vi "generate_zernike_tilt_vectors.vi"(1 "Transform":T1, 2 "Number of modes":i32=12, 3 "Positions on back aperture":cluster{dbl, dbl}[][](array[cluster])) -> (0 "Tilt Vectors":dbl[][](array[numeric]))   [LabVIEW 2010]
uses:
  <vilib>/Analysis/Matrix/Datatypes/RealMatrix.ctl
  <vilib>/Analysis/baseanly.llb/A x Vector.vi
  <vilib>/Analysis/NI_AALBase.lvlib
  <vilib>/Analysis/Matrix/NI_Matrix.lvlib
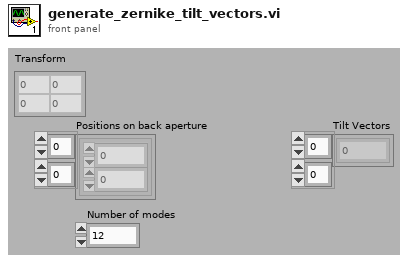
[diagram p1: front panel]
types:
  T1 = typedef "NI_Matrix.lvlib/RealMatrix.ctl" = dbl[][]
  T2 = cluster{"A x Vector[0]":dbl, "A x Vector[1]":dbl}
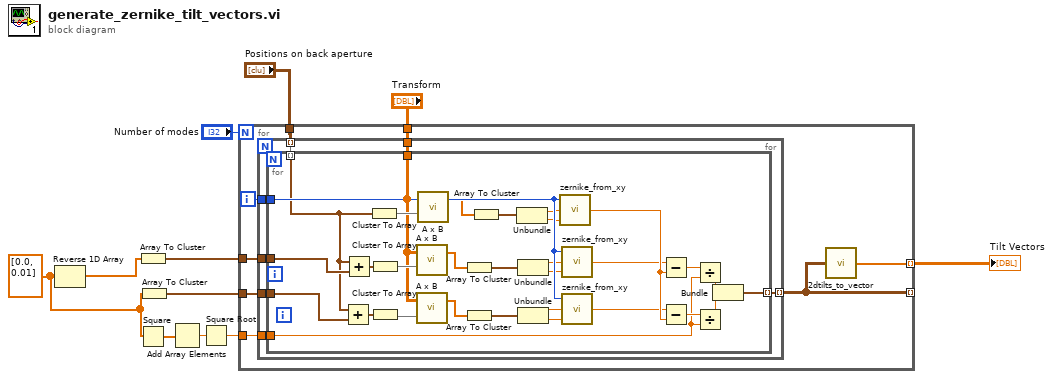
[diagram p0: block diagram]
diagram:
  w2 = dbl[] [0.0, 0.01]
  n1 = Reverse 1D Array(array=w2) -> (reversed array=w3:dbl[])
  n2 = Array To Cluster(array=w3) -> (cluster=w8:cluster{"[0]":dbl, "[1]":dbl})
  n3 = Square(x=w2) -> (x^2=w6:dbl[])
  n4 = Array To Cluster(array=w2) -> (cluster=w7:cluster{"[0]":dbl, "[1]":dbl})
  n5 = Add Array Elements(numeric array=w6) -> (sum=w5:dbl)
  n6 = Square Root(x=w5) -> (sqrt(x)=w4:dbl)
  n7 = for {
    N: "Number of modes" -> [_]
    tunnel: "Positions on back aperture" -> [w18]
    tunnel: [w16] -> _ mode=indexing
    tunnel: [w17] -> w11 mode=indexing
    tunnel: w8 -> [w15]
    tunnel: w7 -> [w14]
    tunnel: w4 -> [w13]
    tunnel: "Transform" -> [w12]
    i -> [w19]
    n8 = for {
      tunnel: w19 -> [w26]
      tunnel: w18 -> [w25] mode=indexing
      tunnel: [w24] -> w16 mode=indexing
      tunnel: w15 -> [w23]
      tunnel: w14 -> [w22]
      tunnel: w13 -> [w21]
      tunnel: w12 -> [w20]
      n9 = for {
        tunnel: w26 -> [w57]
        tunnel: w25 -> [w31] mode=indexing
        tunnel: [w47] -> w24 mode=indexing
        tunnel: w23 -> [w41]
        tunnel: w22 -> [w42]
        tunnel: w21 -> [w40]
        tunnel: w20 -> [w27]
        n10 = Add(x=w31, y=w42) -> (x+y=w32:cluster{dbl, dbl})
        n11 = Add(x=w31, y=w41) -> (x+y=w39:cluster{dbl, dbl})
        n12 = Cluster To Array(cluster=w31) -> (array=w30:dbl[])
        n13 = Cluster To Array(cluster=w39) -> (array=w37:dbl[])
        n14 = Cluster To Array(cluster=w32) -> (array=w35:dbl[])
        n15 = call-poly <vilib>:"A x B.vi"("Vector"=w37, "A"=w27) -> ("A x Vector"=w36:dbl[])  [unwired: 1 out]
        n16 = call-poly <vilib>:"A x B.vi"("Vector"=w35, "A"=w27) -> ("A x Vector"=w34:dbl[])  [unwired: 1 out]
        n17 = call-poly <vilib>:"A x B.vi"("Vector"=w30, "A"=w27) -> ("A x Vector"=w29:dbl[])  [unwired: 1 out]
        n18 = Array To Cluster(array=w36) -> (cluster=w38:T2)
        n19 = Array To Cluster(array=w34) -> (cluster=w33:T2)
        n20 = Array To Cluster(array=w29) -> (cluster=w28:T2)
        n21 = Unbundle(w28) -> ("A x Vector[0]"=w55:dbl, "A x Vector[1]"=w56:dbl)
        n22 = Unbundle(w38) -> ("A x Vector[0]"=w43:dbl, "A x Vector[1]"=w46:dbl)
        n23 = Unbundle(w33) -> ("A x Vector[0]"=w45:dbl, "A x Vector[1]"=w44:dbl)
        n24 = call "zernike_from_xy.vi"("y (-.5 to .5)"=w56, "x (-.5 to .5)"=w55, "Numeric"=w57) -> ("z"=w54:dbl)
        n25 = call "zernike_from_xy.vi"("y (-.5 to .5)"=w46, "x (-.5 to .5)"=w43, "Numeric"=w57) -> ("z"=w53:dbl)
        n26 = call "zernike_from_xy.vi"("y (-.5 to .5)"=w44, "x (-.5 to .5)"=w45, "Numeric"=w57) -> ("z"=w52:dbl)
        n27 = Subtract(x=w53, y=w54) -> (x-y=w51:dbl)
        n28 = Subtract(x=w52, y=w54) -> (x-y=w50:dbl)
        n29 = Divide(x=w51, y=w40) -> (x/y=w49:dbl)
        n30 = Divide(x=w50, y=w40) -> (x/y=w48:dbl)
        n31 = Bundle(w49, w48) -> (w47:cluster{dbl, dbl})  [unwired: 1 out]
      }
    }
    n32 = call "2dtilts_to_vector.vi"("Array"=w16) -> ("Position"=w17:dbl[])
  }
  "Tilt Vectors" <- w11
